vi "Read Data.vi"(8 "AI Rate":dbl=10000.0 format="%.2f", 9 "AI Buffer Size (s)":i32=10, 10 "AI Block Size":i32=5000, 11 "AI task":refnum<k21>[](array[refnum])=["", ""]) -> (1 "Backlog":u8(slide) scale=0.0..100.0, 2 "Input Signals":dbl[][](array[numeric]))   [LabVIEW 2013, in "Lock-In Variable Channels_2.lvclass"]
uses:
  Variable Channel O.O.P/Lock-In Variable Channels_2.lvclass
  <vilib>/DAQmx/read.llb/DAQmx Read (Analog 2D DBL NChan NSamp).vi
  <vilib>/DAQmx/miscellaneous.llb/DAQmx Fill In Error Info.vi
  <resource>/objmgr/daqmx.rc
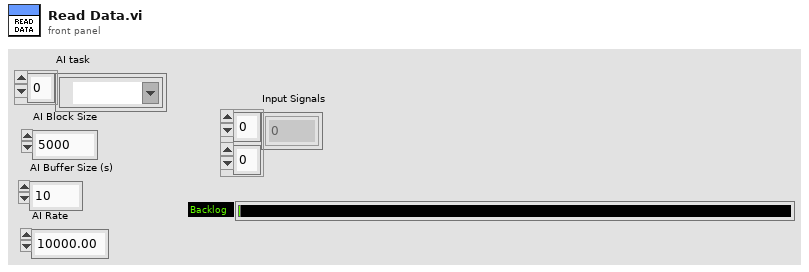
[diagram p1: front panel]
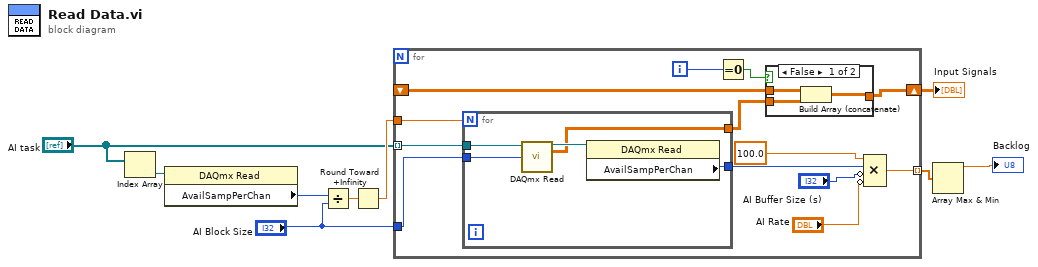
[diagram p0: block diagram]
diagram:
  n1 = Index Array(array="AI task") -> (element=w7:refnum<k21>)  [unwired: 1 in]
  n2 = property class="DAQmx Read"(reference=w7) -> ("AvailSampPerChan"=w6:u32)  [unwired: 1 in, 2 out]
  n3 = Divide(x=w6, y="AI Block Size") -> (x/y=w5:dbl)
  n4 = Round Toward +Infinity(x=w5) -> (ceil(x): smallest int >= x=w4:dbl)
  n5 = for {
    tunnel: "AI task" -> [w14] mode=indexing
    tunnel: [w20] -> w9 mode=indexing
    shift-right: [w15] -> w2
    shift-left: _ -> [w17]
    tunnel: w4 -> [w13]
    tunnel: "AI Block Size" -> [w12]
    i -> [w18]
    n6 = for {
      N: w13 -> [_]
      tunnel: [w30] -> w16
      tunnel: [w29] -> w22
      tunnel: w14 -> [w28]
      tunnel: w12 -> [w27]
      n7 = call-poly <vilib>:"DAQmx Read.vi"("task/channels in"=w28, "number of samples per channel"=w27) -> ("task out"=w31:refnum<k21>, "data"=w30:dbl[][])  [unwired: 11 in, 1 out]
      n8 = property class="DAQmx Read"(reference=w31) -> ("AvailSampPerChan"=w29:u32)  [unwired: 1 in, 2 out]
    }
    n9 = Equal To 0?(x=w18) -> (x = 0?=w19:bool)
    n10 = case shown="False" w19 {
      tunnel: w17 -> [w23 _]
      tunnel: w16 -> [w25 w26]
      tunnel: [w24 w26] -> w15
      frame False {
        n11 = Build Array (concatenate)(w23, w25) -> (w24:dbl[][])
      }
      frame True {
      }
    }
    n12 = Compound Arithmetic op=MULTIPLY(100.0 ("value"), w22, invert "AI Buffer Size (s)", invert "AI Rate") -> (w20:dbl)
  }
  "Input Signals" <- w2
  n13 = Array Max & Min(array=w9) -> (max value=→"Backlog":dbl)  [unwired: 3 out]
